vi "liberaToCmd.vi"(4 "Set Environment":T1, 5 "value":string, 6 "loops":i32=1, 7 "acquire time":u32, 8 "samples":u32=1, 9 "triggered":bool, 10 "decimated":bool, 11 "cmd":T2(ring)=enum."acquireStream") -> (0 "jsonargs":string, 3 "cmd":string)   [LabVIEW 2012]
uses:
  libera_env.ctl
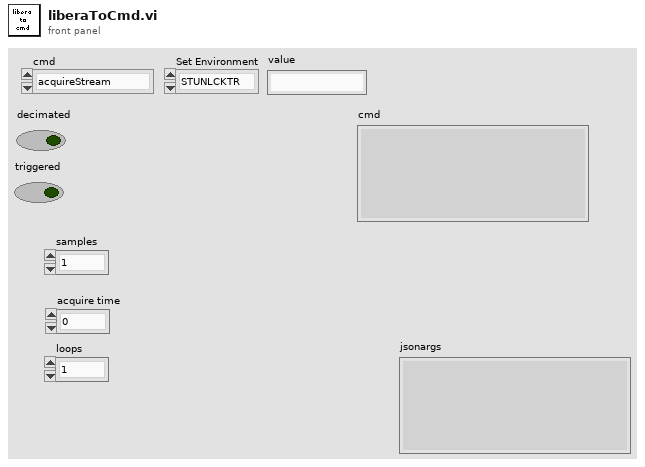
[diagram p1: front panel]
types:
  T1 = typedef "libera_env.ctl" = enum16{"STUNLCKTR", "MTSYNCIN", "MTUNLCKTR", "MTNCOSHFT", "MTVCXOFFS", "POLYPHASE_FIR", "NOTCH2", "NOTCH1", "DDC_MAFDELAY", "DDC_MAFLENGTH", "SWDELAY", "EXTSWITCH", "TRIGDELAY", "PMDEC", "PMOFFSET", "ILKSTATUS", "ILK", "DSC", "AGC", "GAIN", "SWITCH", "QOFFSET", "YOFFSET", "XOFFSET", "KY", "KX"}
  T2 = enum16{"setEnv", "stopAcquire", "setTime", "acquireAVG", "acquireADCSP", "acquireADCCW", "acquireStream", "acquireDD"}
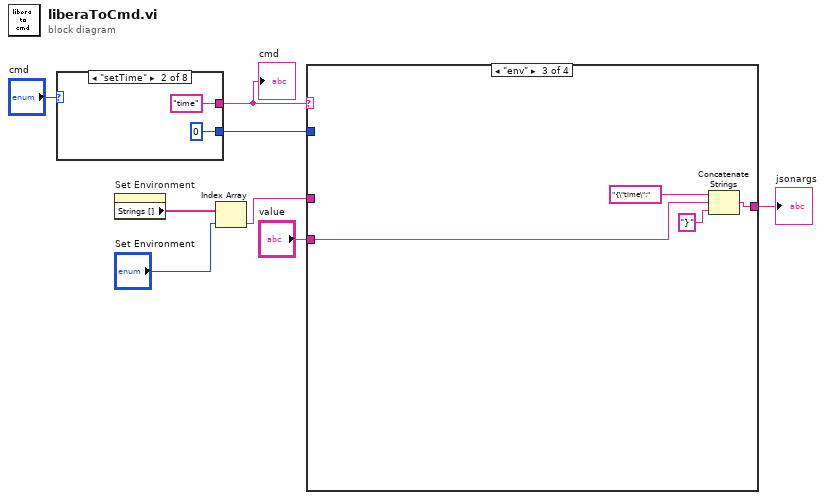
[diagram p0: block diagram]
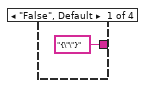
[diagram p2: hidden frame]
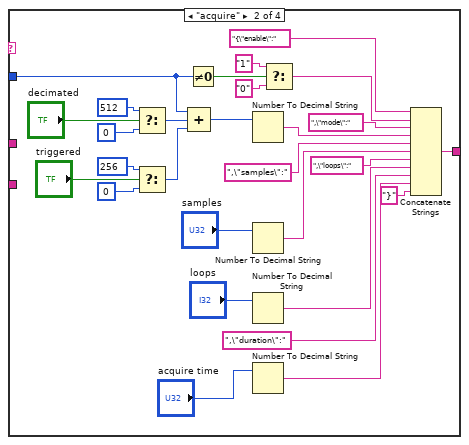
[diagram p3: hidden frame]
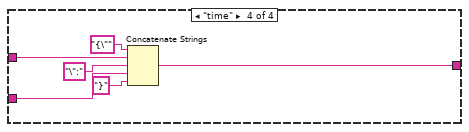
[diagram p4: hidden frame]
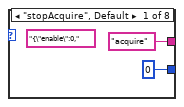
[diagram p5: hidden frame]
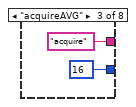
[diagram p6: hidden frame]
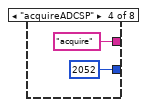
[diagram p7: hidden frame]
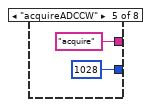
[diagram p8: hidden frame]
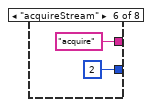
[diagram p9: hidden frame]
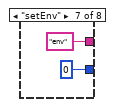
[diagram p10: hidden frame]
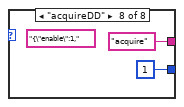
[diagram p11: hidden frame]
diagram:
  n1 = case shown="\"setTime\"" "cmd" {
    tunnel: ["acquire" "time" "acquire" "acquire" "acquire" "acquire" "env" "acquire"] -> w6
    tunnel: [u32 0 ("f") u32 0 ("f") u32 16 u32 2052 u32 1028 u32 2 u32 0 u32 1] -> w5
    frame "stopAcquire", Default {
      (unwired) "{\"enable\":0,"
    }
    frame "setTime" {
    }
    frame "acquireAVG" {
    }
    frame "acquireADCSP" {
    }
    frame "acquireADCCW" {
    }
    frame "acquireStream" {
    }
    frame "setEnv" {
    }
    frame "acquireDD" {
      (unwired) "{\"enable\":1,"
    }
  }
  "cmd" <- w6
  n2 = property on="Set Environment" class="Enum (strict)"() -> ("Strings []"=w4:string[])  [unwired: 2 in, 2 out]
  n3 = Index Array(array=w4, index="Set Environment") -> (element=w2:string)
  n4 = case shown="\"env\"" w6 {
    tunnel: ["{\"\"}" w40 w54 w58] -> w7
    tunnel: w5 -> [_ w30 _ _]
    tunnel: w2 -> [_ _ _ w62]
    tunnel: "value" -> [_ _ w56 w60]
    frame "False", Default {
    }
    frame "acquire" {
      n5 = Select(t=u32 512, s="decimated", f=u32 0) -> (s? t:f=w34:u32)
      n6 = Select(t=u32 256, s="triggered", f=u32 0) -> (s? t:f=w33:u32)
      n7 = Not Equal To 0?(x=w30) -> (x != 0?=w29:bool)
      n8 = Compound Arithmetic op=ADD(w30, w34, w33) -> (w53:u32)
      n9 = Number To Decimal String(number=w53) -> (decimal integer string=w51:string)  [unwired: 1 in]
      n10 = Number To Decimal String(number="samples") -> (decimal integer string=w48:string)  [unwired: 1 in]
      n11 = Number To Decimal String(number="loops") -> (decimal integer string=w45:string)  [unwired: 1 in]
      n12 = Number To Decimal String(number="acquire time") -> (decimal integer string=w42:string)  [unwired: 1 in]
      n13 = Select(t="1", s=w29, f="0") -> (s? t:f=w26:string)
      n14 = Concatenate Strings("{\"enable\":", w26, ",\"mode\":" ("string"), w51, ",\"samples\":" ("string"), w48, ",\"loops\":" ("string"), w45, ",\"duration\":" ("string"), w42, "}" ("string")) -> (w40:string)
    }
    frame "env" {
      n15 = Concatenate Strings("{\"time\":" ("string"), w56, "}" ("string")) -> (w54:string)
    }
    frame "time" {
      n16 = Concatenate Strings("{\"" ("string"), w62, "\":" ("string"), w60, "}" ("string")) -> (w58:string)
    }
  }
  "jsonargs" <- w7
